vi "Update Game Board Component.vi"(11 "Game Board in":refnum<class "Game Board.lvclass">) -> (3 "Game Board out":refnum<class "Game Board.lvclass">)   [LabVIEW 2024, in "Game Board.lvclass"]
doc: "MIT Licence\nCopyright (c) 2024 David Grollier"
uses:
  Game Board.lvclass
  Game Board.lvclass/Game Board.ctl
  Game Board Component/Movable/Movable.lvclass
  Game Board Component/Game Board Component.lvclass
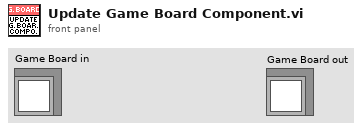
[diagram p1: front panel]
types:
  T1 = map{string, refnum<class "Game Board Component.lvclass">}
  T2 = cluster{"Name":string, "Game Board Component":refnum<class "Game Board Component.lvclass">}
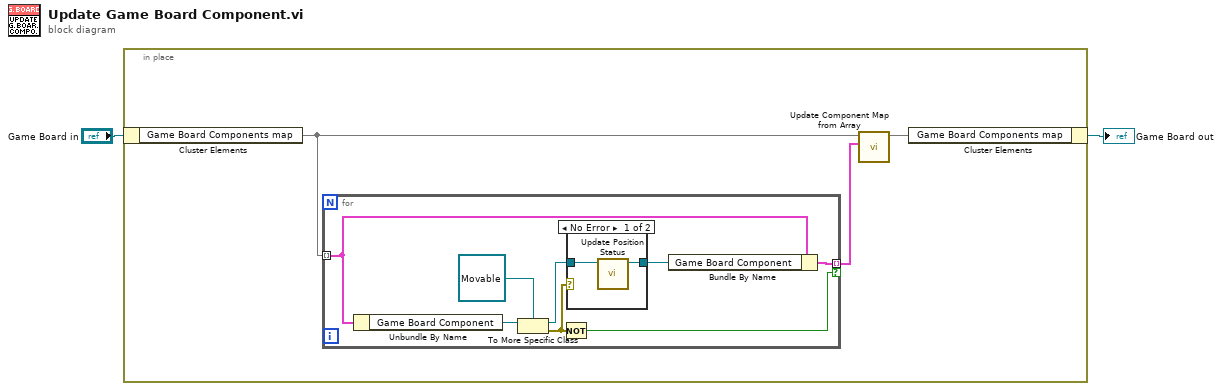
[diagram p0: block diagram]
diagram:
  n1 = in-place {
    n2 = in-place-cluster #1("Game Board in") -> ("Game Board Components map"=w4:T1)
    n3 = for {
      tunnel: w4 -> [w11] mode=indexing
      tunnel: [w10] -> w5 mode=indexing if=w9
      n4 = Unbundle By Name(w11) -> ("Game Board Component"=w12:refnum<class "Game Board Component.lvclass">)
      n5 = To More Specific Class(target class=refnum<class "Movable.lvclass"> refnum ("Movable in"), reference=w12) -> (specific class reference=w8:refnum<class "Movable.lvclass">, error out=w6:errorcluster)  [unwired: 1 in]
      n6 = Not(x=w6) -> (.not. x?=w9:bool)
      n7 = case shown="No Error" w6 {
        tunnel: w8 -> [w15 w16]
        tunnel: [w14 w16] -> w7
        frame No Error {
          n8 = call "Update Position Status.vi"("Movable in"=w15) -> ("Movable out"=w14:refnum<class "Movable.lvclass">)  [unwired: 10 in]
        }
        frame Error {
        }
      }
      n9 = Bundle By Name(cluster=w11, "Game Board Component"=w7) -> (w10:T2)
    }
    n10 = call "Update Component Map from Array.vi"("Array of components in"=w5, "Game Board Components[] in"=w4) -> ("Game Board Components[] out"=w3:T1)  [unwired: 9 in]
    n11 = in-place-cluster #1("Game Board Components map"=w3) -> (→"Game Board out":refnum<class "Game Board.lvclass">)
  }
